vi "ROS_Master_CleanNodes.vi"(3 "ROS_Master in":T1) -> (1 "ROS_Master out":T1)   [LabVIEW 2012]
doc: "Removes a closed topic or service from the globals"
uses:
  ROS_Topic.ctl
  ROS_Node.ctl
  ROS_Service.ctl
  ROS_Master.ctl
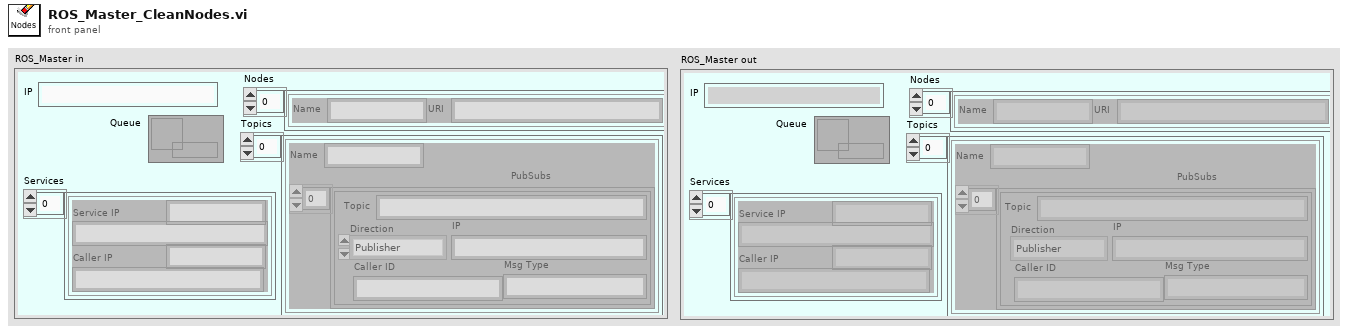
[diagram p1: front panel]
types:
  T1 = typedef "ROS_Master.ctl" = cluster{"IP":string, "Topics":cluster{"Name":string, "PubSubs":T2[]}[], "Nodes":T3[], "Services":T4[], "Queue":refnum<queue>}
  T2 = typedef "ROS_Topic.ctl" = cluster{"Caller ID":string, "IP":string, "Msg Type":string, "Direction":enum16{"Publisher", "Subscriber"}, "Topic":string}
  T3 = typedef "ROS_Node.ctl" = cluster{"Name":string, "URI":string}
  T4 = typedef "ROS_Service.ctl" = cluster{"Service":string, "Service IP":string, "Caller IP":string, "Caller ID":string}
  T5 = cluster{"Caller ID":string, "Caller IP":string}[]
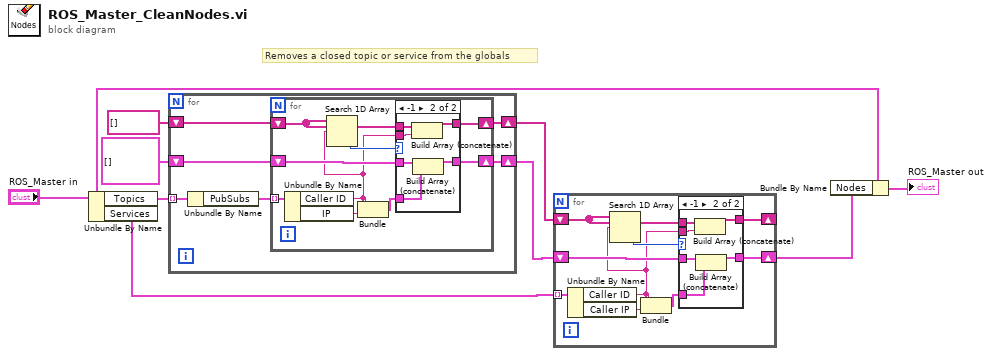
[diagram p0: block diagram]
diagram:
  # "Removes a closed topic or service from the globals"
  n1 = Unbundle By Name("ROS_Master in") -> ("Topics"=w9:cluster{"Name":string, "PubSubs":T2[]}[], "Services"=w6:T4[])
  n2 = for {
    tunnel: w9 -> [w15] mode=indexing
    shift-right: [w12] -> w5
    shift-left: cluster{"Caller ID":string, "IP":string}[] [] -> [w13]
    shift-right: [w11] -> w4
    shift-left: string[] [] -> [w10]
    n3 = Unbundle By Name(w15) -> ("PubSubs"=w14:T2[])
    n4 = for {
      tunnel: w14 -> [w24] mode=indexing
      shift-right: [w23] -> w12
      shift-left: w13 -> [w22]
      shift-right: [w19] -> w11
      shift-left: w10 -> [w18]
      n5 = Unbundle By Name(w24) -> ("Caller ID"=w16:string, "IP"=w21:string)
      n6 = Search 1D Array(1D array=w18, element=w16) -> (index of element=w17:i32)  [unwired: 1 in]
      n7 = Bundle("Caller ID"=w16, "IP"=w21) -> (w20:cluster{"Caller ID":string, "IP":string})  [unwired: 1 in]
      n8 = case shown="-1" w17 {
        tunnel: [w26 w32] -> w23
        tunnel: w20 -> [_ w31]
        tunnel: w22 -> [w26 w30]
        tunnel: w16 -> [_ w29]
        tunnel: [w25 w28] -> w19
        tunnel: w18 -> [w25 w27]
        frame Default {
        }
        frame -1 {
          n9 = Build Array (concatenate)(w27, w29) -> (w28:string[])
          n10 = Build Array (concatenate)(w30, w31) -> (w32:cluster{"Caller ID":string, "IP":string}[])
        }
      }
    }
  }
  n11 = for {
    tunnel: w6 -> [w41] mode=indexing
    shift-right: [w40] -> w3
    shift-left: w5 -> [w39]
    shift-right: [w36] -> _
    shift-left: w4 -> [w35]
    n12 = Unbundle By Name(w41) -> ("Caller ID"=w33:string, "Caller IP"=w38:string)
    n13 = Search 1D Array(1D array=w35, element=w33) -> (index of element=w34:i32)  [unwired: 1 in]
    n14 = Bundle("Caller ID"=w33, "Caller IP"=w38) -> (w37:cluster{"Caller ID":string, "Caller IP":string})  [unwired: 1 in]
    n15 = case shown="-1" w34 {
      tunnel: [w43 w49] -> w40
      tunnel: w37 -> [_ w48]
      tunnel: w39 -> [w43 w47]
      tunnel: w33 -> [_ w46]
      tunnel: [w42 w45] -> w36
      tunnel: w35 -> [w42 w44]
      frame Default {
      }
      frame -1 {
        n16 = Build Array (concatenate)(w44, w46) -> (w45:string[])
        n17 = Build Array (concatenate)(w47, w48) -> (w49:T5)
      }
    }
  }
  n18 = Bundle By Name(cluster="ROS_Master in", "Nodes"=w3) -> (→"ROS_Master out":T1)
